vi "Vision Tracking Drive Control.vi"(11 "Cluster in":T11) -> (3 "Cluster out":T11)   [LabVIEW 2018]
uses:
  <vilib>/Rock Robotics/WPI/Joystick/WPI_JoystickDevRef.ctl
  <vilib>/Rock Robotics/WPI/Joystick/WPI_JoystickDeviceEnum.ctl
  <vilib>/Rock Robotics/WPI/DriverStation/WPI_DriverStationRobotMode2.ctl
  <vilib>/Rock Robotics/WPI/RobotDrive/WPI_RobotDriveDevRef.ctl
  <vilib>/Rock Robotics/WPI/MotorControl/WPI_MotorControlDeviceRef.ctl
  <vilib>/Rock Robotics/WPI/MotorControl/WPI_MotorControlType.ctl
  <vilib>/Rock Robotics/SystemInterfaces/DIO/FPGA_DIOPWMChannel.ctl
  <vilib>/Rock Robotics/WPI/PWM/WPI_PWMDeadband.ctl
  <vilib>/Rock Robotics/SystemInterfaces/DIO/FPGA_DIOChannel.ctl
  Vision States.ctl
  <vilib>/Rock Robotics/WPI/ThirdParty/Phoenix-LabVIEW/Motor Controller/Controls/CTRE_Phoenix_MotorControl_ControlMode.ctl
  <vilib>/Rock Robotics/Network Tables/NT Read Number.vi
  Robot Global Data.vi
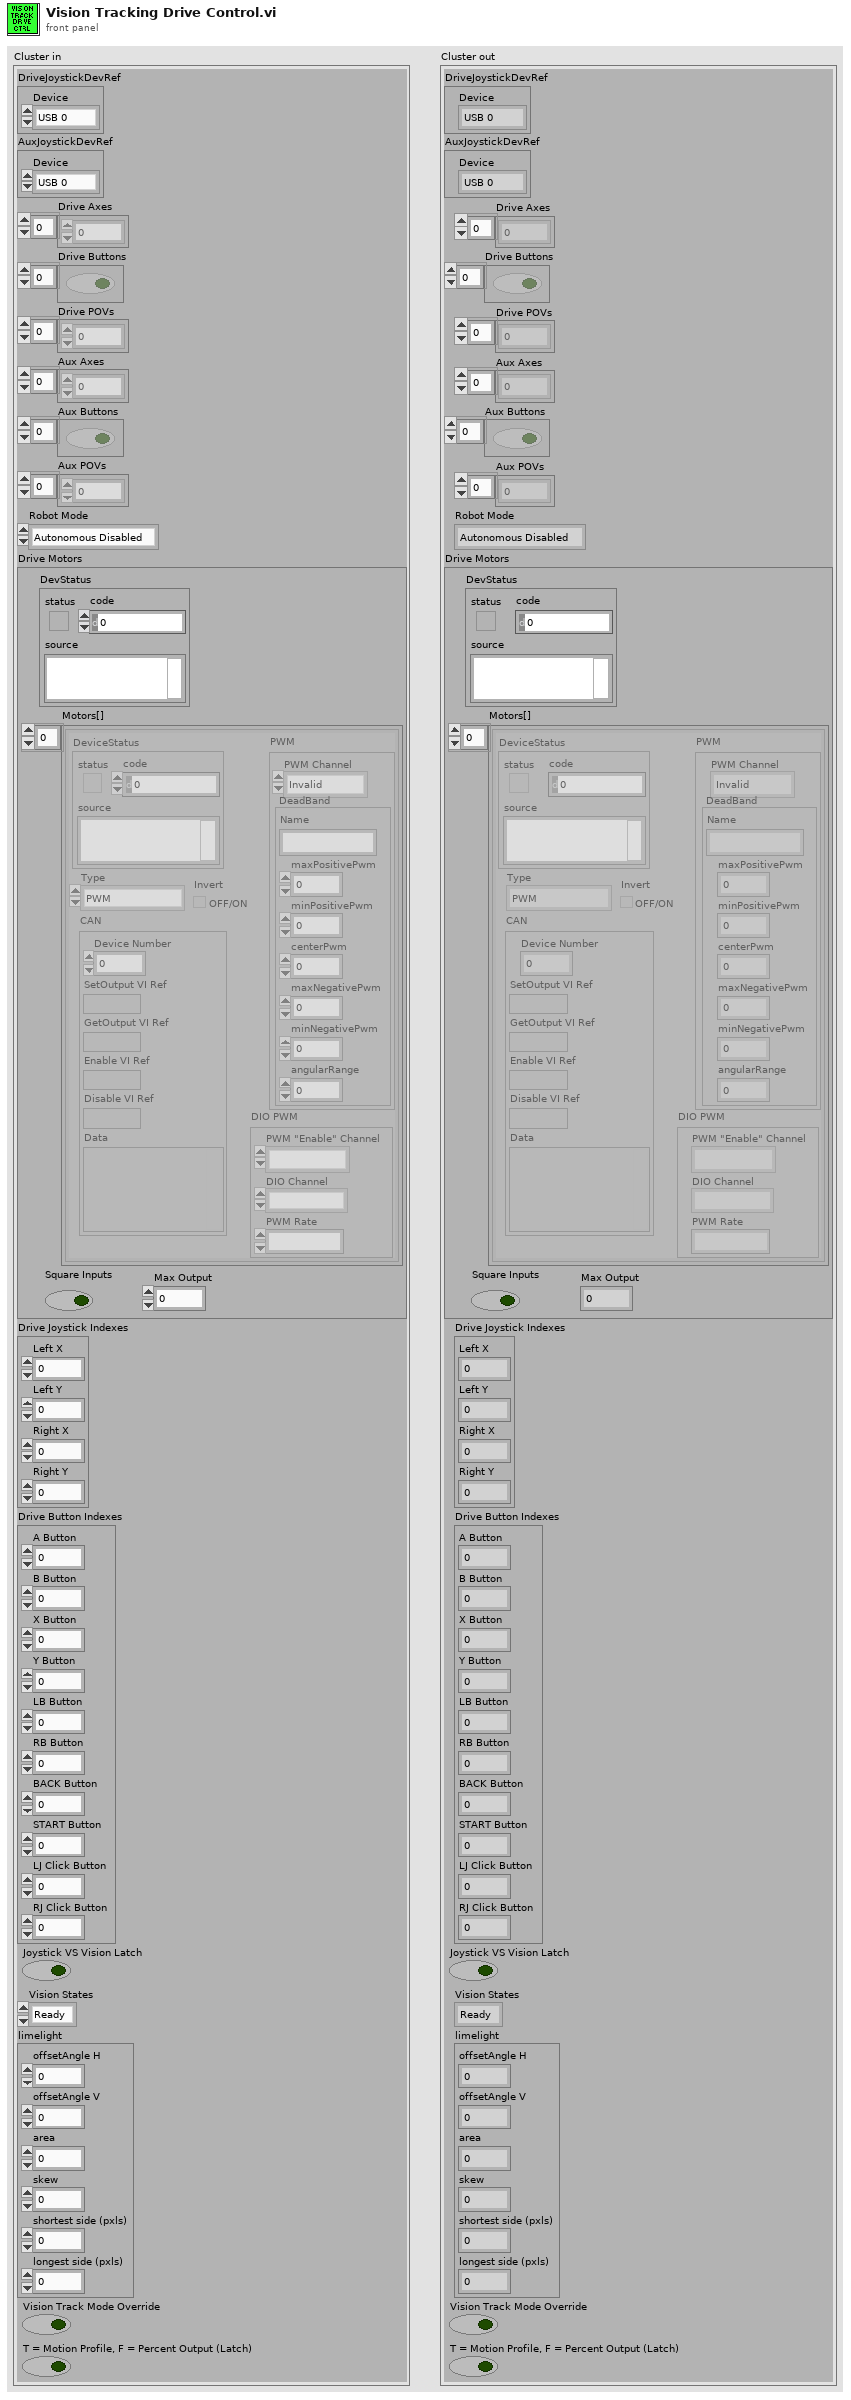
[diagram p1: front panel]
types:
  T1 = typedef "WPI_JoystickDevRef.ctl" = cluster{"Device":T2}
  T2 = typedef "WPI_JoystickDeviceEnum.ctl" = enum16{"USB 0", "USB 1", "USB 2", "USB 3", "USB 4", "USB 5"}
  T3 = typedef "WPI_DriverStationRobotMode2.ctl" = enum16{"Autonomous Disabled", "Autonomous Enabled", "Teleop Disabled", "Teleop Enabled", "Disconnected", "Finish", "Test Disabled", "Test Enabled", "Emergency Stopped"}
  T4 = typedef "WPI_RobotDriveDevRef.ctl" = cluster{"DevStatus":errorcluster, "Motors[]":T5[], "Square Inputs":bool, "Max Output":dbl}
  T5 = typedef "WPI_MotorControlDeviceRef.ctl" = cluster{"DeviceStatus":errorcluster, "Type":T6, "PWM":cluster{"PWM Channel":T7, "DeadBand":T8}, "CAN":cluster{"Device Number":u8, "SetOutput VI Ref":variant, "GetOutput VI Ref":variant, "Enable VI Ref":variant, "Disable VI Ref":variant, "Data":variant}, "Invert":bool, "DIO PWM":cluster{"PWM \"Enable\" Channel":T7, "DIOChannel":T9, "PWM Rate":dbl}}
  T6 = typedef "WPI_MotorControlType.ctl" = enum16{"PWM", "CAN", "DIO PWM"}
  T7 = typedef "FPGA_DIOPWMChannel.ctl" = enum8{"PWM 0", "PWM 1", "PWM 2", "PWM 3", "PWM 4", "PWM 5", "PWM 6", "PWM 7", "PWM 8", "PWM 9", "PWM MXP 0", "PWM MXP 1", "PWM MXP 2", "PWM MXP 3", "PWM MXP 4", "PWM MXP 5", "PWM MXP 6", "PWM MXP 7", "PWM MXP 8", "PWM MXP 9", "Invalid"}
  T8 = typedef "WPI_PWMDeadband.ctl" = cluster{"Name":string, "maxPositivePwm":i32, "minPositivePwm":i32, "centerPwm":i32, "maxNegativePwm":i32, "minNegativePwm":i32, "angularRange":u16}
  T9 = typedef "FPGA_DIOChannel.ctl" = enum8{"DIO 0", "DIO 1", "DIO 2", "DIO 3", "DIO 4", "DIO 5", "DIO 6", "DIO 7", "DIO 8", "DIO 9", "DIO MXP 0", "DIO MXP 1", "DIO MXP 2", "DIO MXP 3", "DIO MXP 4", "DIO MXP 5", "DIO MXP 6", "DIO MXP 7", "DIO MXP 8", "DIO MXP 9", "DIO MXP 10", "DIO MXP 11", "DIO MXP 12", "DIO MXP 13", "DIO MXP 14", "DIO MXP 15", "SPI Port CS1", "SPI Port CS2", "SPI Port CS3", "SPI Port MISO", "SPI Port MOSI", "Invalid"}
  T10 = typedef "Vision States.ctl" = enum16{"Ready", "Forward Until Target at Edge", "Vision Track"}
  T11 = cluster{"DriveJoystickDevRef":T1, "AuxJoystickDevRef":T1, "Drive Axes":dbl[], "Drive Buttons":bool[], "Drive POVs":i16[], "Aux Axes":dbl[], "Aux Buttons":bool[], "Aux POVs":i16[], "Robot Mode":T3, "Drive Motors":T4, "Drive Joystick Indexes":cluster{"Left X":i32, "Left Y":i32, "Right X":i32, "Right Y":i32}, "Drive Button Indexes":cluster{"A Button":i32, "B Button":i32, "X Button":i32, "Y Button":i32, "LB Button":i32, "RB Button":i32, "BACK Button":i32, "START Button":i32, "LJ Click Button":i32, "RJ Click Button":i32}, "Joystick VS Vision Latch":bool, "Vision States":T10, "limelight":cluster{"offsetAngle H":dbl, "offsetAngle V":dbl, "area":dbl, "skew":dbl, "shortest side (pxls)":dbl, "longest side (pxls)":dbl}, "Vision Track Mode Override":bool, "T = Motion Profile, F = Percent Output (Latch)":bool}
  T12 = typedef "Which Robot Enum.ctl" = enum16{"Competition Bot", "Practice Bot", "Code Bot"}
  T13 = typedef "CTRE_Phoenix_MotorControl_ControlMode.ctl" = u16
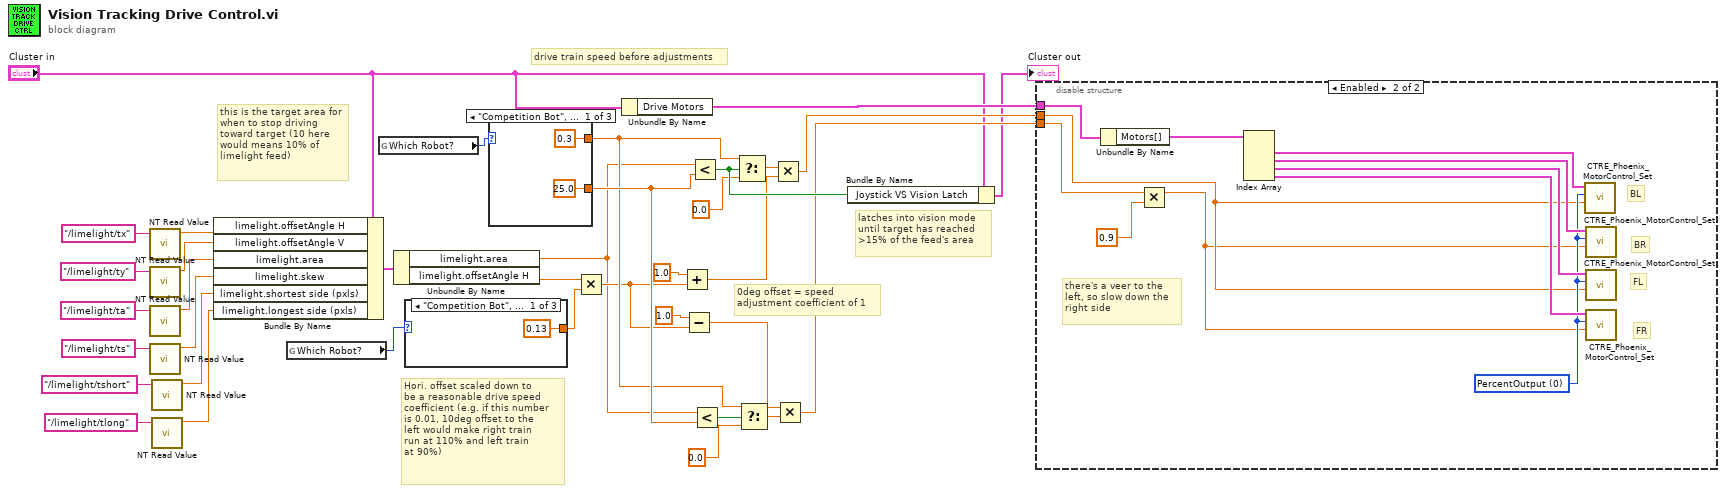
[diagram p0: block diagram]
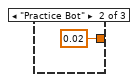
[diagram p2: hidden frame]
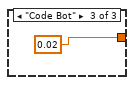
[diagram p3: hidden frame]
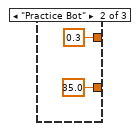
[diagram p4: hidden frame]
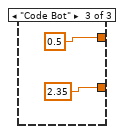
[diagram p5: hidden frame]
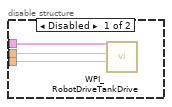
[diagram p6: hidden frame]
diagram:
  # "latches into vision mode \nuntil target has reached \n>15% of the feed's area"
  # "drive train speed before adjustments"
  # "this is the target area for\nwhen to stop driving \ntoward target (10 here \nwould means 10% of \nlimelight feed)"
  # "Hori. offset scaled down to\nbe a reasonable drive speed\ncoefficient (e.g. if this number\nis 0.01, 10deg offset to the \nleft would make right train \nrun at 110% and left train \nat 90%)"
  # "0deg offset = speed \nadjustment coefficient of 1"
  n1 = call-poly <vilib>:"NT Read Value.vi"("Name"="/limelight/tx") -> ("Numeric"=w9:dbl)  [unwired: 9 in, 1 out]
  n2 = call-poly <vilib>:"NT Read Value.vi"("Name"="/limelight/ty") -> ("Numeric"=w10:dbl)  [unwired: 9 in, 1 out]
  n3 = call-poly <vilib>:"NT Read Value.vi"("Name"="/limelight/ta") -> ("Numeric"=w11:dbl)  [unwired: 9 in, 1 out]
  n4 = call-poly <vilib>:"NT Read Value.vi"("Name"="/limelight/ts") -> ("Numeric"=w12:dbl)  [unwired: 9 in, 1 out]
  n5 = call-poly <vilib>:"NT Read Value.vi"("Name"="/limelight/tshort") -> ("Numeric"=w35:dbl)  [unwired: 9 in, 1 out]
  n6 = call-poly <vilib>:"NT Read Value.vi"("Name"="/limelight/tlong") -> ("Numeric"=w36:dbl)  [unwired: 9 in, 1 out]
  n7 = Bundle By Name(cluster="Cluster in", "limelight.offsetAngle H"=w9, "limelight.offsetAngle V"=w10, "limelight.area"=w11, "limelight.skew"=w12, "limelight.shortest side (pxls)"=w35, "limelight.longest side (pxls)"=w36) -> (w13:T11)
  n8 = global read "Robot Global Data.vi" "Which Robot?"() -> (w1:T12)
  n9 = global read "Robot Global Data.vi" "Which Robot?"() -> (w2:T12)
  n10 = Unbundle By Name(w13) -> ("limelight.area"=w24:dbl, "limelight.offsetAngle H"=w16:dbl)
  n11 = case shown="\"Competition Bot\", Default" w1 {
    tunnel: [0.13 ("y") 0.02 ("y") 0.02 ("y")] -> w17
    frame "Competition Bot", Default {
    }
    frame "Practice Bot" {
    }
    frame "Code Bot" {
    }
  }
  n12 = case shown="\"Competition Bot\", Default" w2 {
    tunnel: [25.0 35.0 2.35] -> w30
    tunnel: [0.3 ("t") 0.3 ("t") 0.5 ("t")] -> w29
    frame "Competition Bot", Default {
    }
    frame "Practice Bot" {
    }
    frame "Code Bot" {
    }
  }
  n13 = Multiply(x=w16, y=w17) -> (x*y=w27:dbl)
  n14 = Unbundle By Name("Cluster in") -> ("Drive Motors"=w31:T4)
  n15 = Add(x=1.0, y=w27) -> (x+y=w21:dbl)
  n16 = Subtract(x=1.0, y=w27) -> (x-y=w28:dbl)
  n17 = Less?(x=w24, y=w30) -> (x < y?=w32:bool)
  n18 = Less?(x=w24, y=w30) -> (x < y?=w20:bool)
  n19 = Select(t=w29, s=w32, f=0.0) -> (s? t:f=w15:dbl)
  n20 = Select(t=w29, s=w20, f=0.0) -> (s? t:f=w23:dbl)
  n21 = Multiply(x=w15, y=w21) -> (x*y=w18:dbl)
  n22 = Multiply(x=w28, y=w23) -> (x*y=w25:dbl)
  n23 = Bundle By Name(cluster="Cluster in", "Joystick VS Vision Latch"=w32) -> (→"Cluster out":T11)
  n24 = disable-structure shown="Enabled" {
    disable-tunnel: w31 -> [w48 w53]
    disable-tunnel: w25 -> [w47 w51]
    disable-tunnel: w18 -> [w46 w52]
    frame Disabled {
      n25 = call <vilib>:"WPI_RobotDriveTankDrive.vi"("Right axis value"=w47, "Left axis value"=w46, "RobotDriveDevRef"=w48) -> ()  [unwired: 6 in, 3 out]
    }
    frame Enabled {
      w54 = T13 0 items=["PercentOutput"=0, "Position"=1, "Velocity"=2, "Current"=3, "Follower"=5, "MotionProfile"=6, "MotionMagic"=7, "MotionProfileArc"=10, "Disabled"=15] ("Control Mode")
      # "there's a veer to the\nleft, so slow down the\nright side"
      # "FR"
      # "FL"
      # "BR"
      # "BL"
      n26 = Unbundle By Name(w53) -> ("Motors[]"=w59:T5[])
      n27 = Multiply(x=w51, y=0.9) -> (x*y=w50:dbl)
      n28 = Index Array(array=w59) -> (element #1=w58:T5, element #2=w55:T5, element #3=w57:T5, element #4=w56:T5)  [unwired: 4 in]
      n29 = call <vilib>:"CTRE_Phoenix_MotorControl_Set.vi"("Output"=w52, "Control Mode"=w54, "PhoenixMotorControlDevRef"=w58) -> ()  [unwired: 7 in, 2 out]
      n30 = call <vilib>:"CTRE_Phoenix_MotorControl_Set.vi"("Output"=w50, "Control Mode"=w54, "PhoenixMotorControlDevRef"=w55) -> ()  [unwired: 7 in, 2 out]
      n31 = call <vilib>:"CTRE_Phoenix_MotorControl_Set.vi"("Output"=w52, "Control Mode"=w54, "PhoenixMotorControlDevRef"=w57) -> ()  [unwired: 7 in, 2 out]
      n32 = call <vilib>:"CTRE_Phoenix_MotorControl_Set.vi"("Output"=w50, "Control Mode"=w54, "PhoenixMotorControlDevRef"=w56) -> ()  [unwired: 7 in, 2 out]
    }
  }
